vi "ParsesCANFrame.vi"(11 "CAN数据帧数组":T1(array[cluster])) -> (3 "CAN数据帧数组(out)":T1(array[cluster]), 4 "CAN报文显示":string[][](table))   [LabVIEW 2018]
panel:
  in  "空数组":u8[](array[numeric])
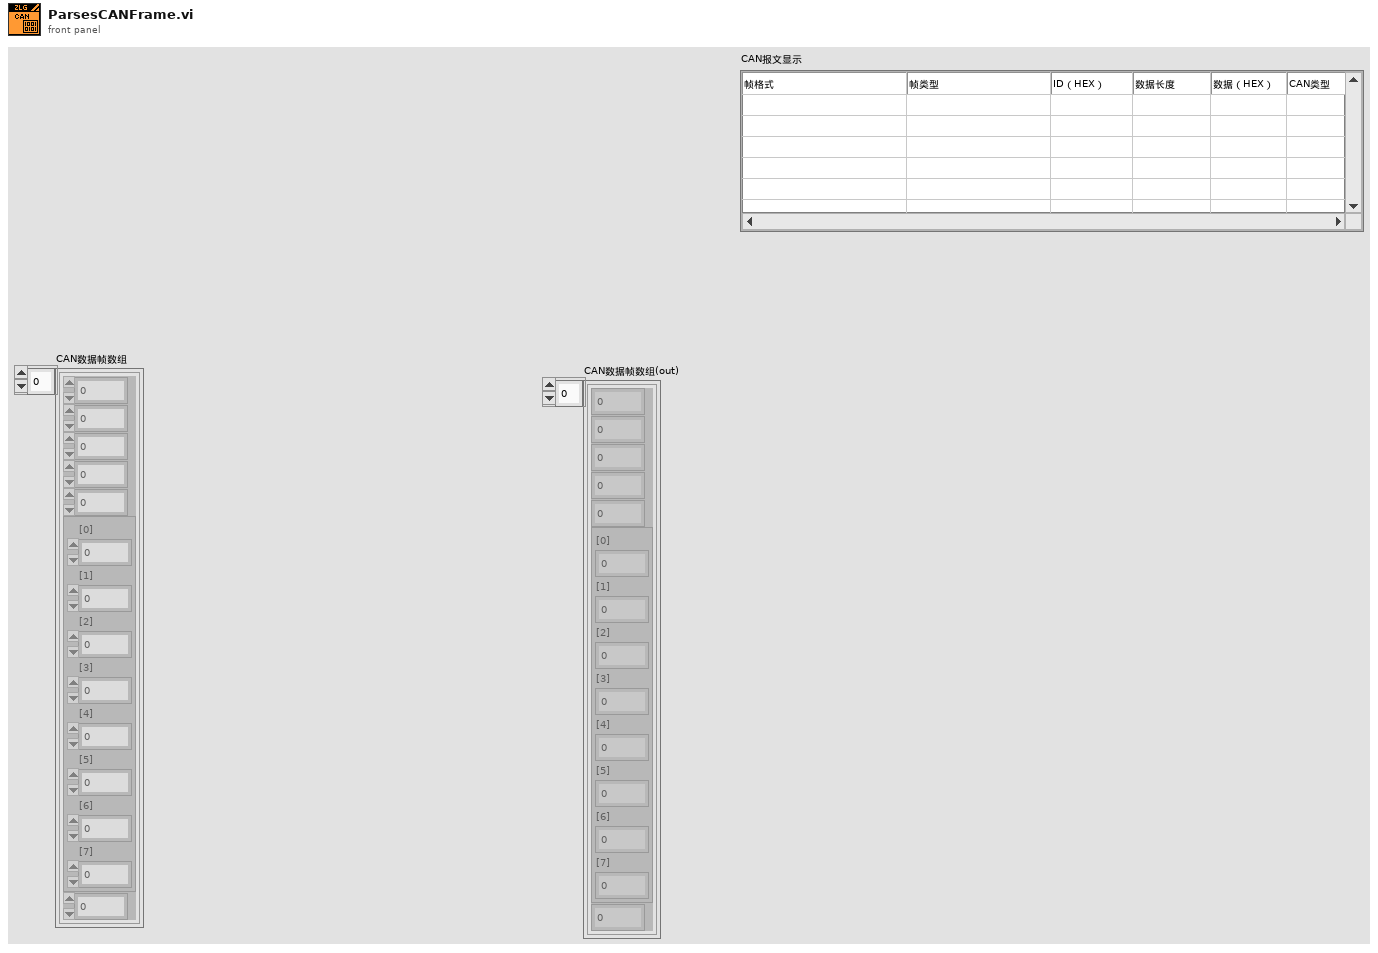
[diagram p1: front panel]
types:
  T1 = cluster{u32, u8, u8, u8, u8, cluster{"[0]":u8, "[1]":u8, "[2]":u8, "[3]":u8, "[4]":u8, "[5]":u8, "[6]":u8, "[7]":u8}, u64}[]
  T2 = cluster{"[0]":u8, "[1]":u8, "[2]":u8, "[3]":u8, "[4]":u8, "[5]":u8, "[6]":u8, "[7]":u8}
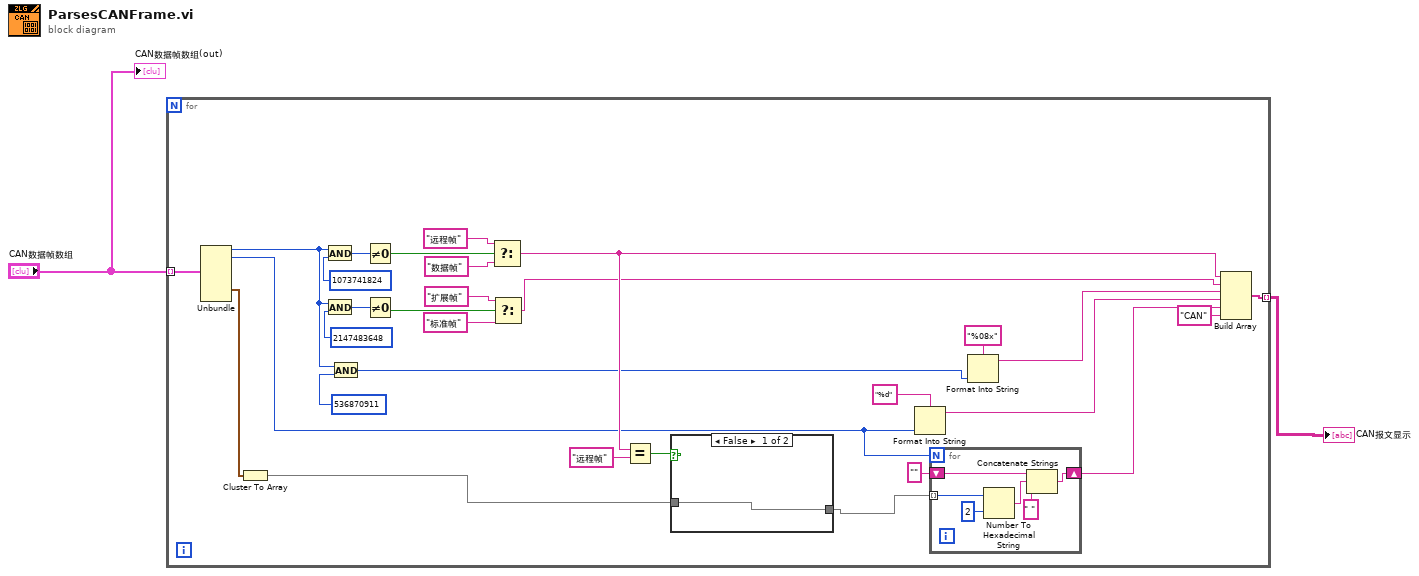
[diagram p0: block diagram]
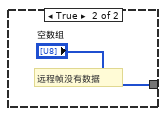
[diagram p2: hidden frame]
diagram:
  n1 = for {
    tunnel: "CAN数据帧数组" -> [w16] mode=indexing
    tunnel: [w9] -> w1 mode=indexing
    n2 = Unbundle(w16) -> (w27:u32, w3:u8, w26:T2)  [unwired: 4 out]
    n3 = Cluster To Array(cluster=w26) -> (array=w17:u8[])
    n4 = And(x=w27, y=u32 1073741824) -> (x .and. y?=w28:u32)
    n5 = And(x=w27, y=u32 2147483648) -> (x .and. y?=w29:u32)
    n6 = And(x=w27, y=u32 536870911) -> (x .and. y?=w5:u32)
    n7 = Not Equal To 0?(x=w28) -> (x != 0?=w21:bool)
    n8 = Not Equal To 0?(x=w29) -> (x != 0?=w20:bool)
    n9 = Select(t="远程帧", s=w21, f="数据帧") -> (s? t:f=w13:string)
    n10 = Select(t="扩展帧", s=w20, f="标准帧") -> (s? t:f=w12:string)
    n11 = Equal?(x=w13, y="远程帧") -> (x = y?=w18:bool)
    n12 = case shown="False" w18 {
      tunnel: [w39 "空数组"] -> w6
      tunnel: w17 -> [w39 _]
      frame False {
      }
      frame True {
        # "远程帧没有数据"
      }
    }
    n13 = Format Into String(format string="%d", w3) -> (resulting string=w10:string)  [unwired: 2 in, 1 out]
    n14 = for {
      N: w3 -> [_]
      shift-right: [w35] -> w4
      shift-left: "" -> [w33]
      tunnel: w6 -> [w34] mode=indexing
      n15 = Number To Hexadecimal String(1:i16 2 ("width (-)"), 2:w34) -> (0:w37:string)
      n16 = Concatenate Strings(w33, w37, " " ("string")) -> (w35:string)
    }
    n17 = Format Into String(format string="%08x", w5) -> (resulting string=w11:string)  [unwired: 2 in, 1 out]
    n18 = Build Array(w13, w12, w11, w10, w4, "CAN" ("元素")) -> (w9:string[])
  }
  "CAN报文显示" <- w1
  "CAN数据帧数组(out)" <- "CAN数据帧数组"
